vi "Cleanup.vi"(8 "error in (no error)":errorcluster, 11 "PlatformConfigPanel in":refnum<class "PlatformConfigPanel.lvclass">) -> (0 "error out":errorcluster)   [LabVIEW 2020, in "PicoG-App.lvlib" / "PlatformConfigPanel.lvclass"]
uses:
  PlatformConfigPanel.lvclass
  <vilib>/IlluminatedG/IG OOPanel/OOPanel/Panel/Panel.lvclass
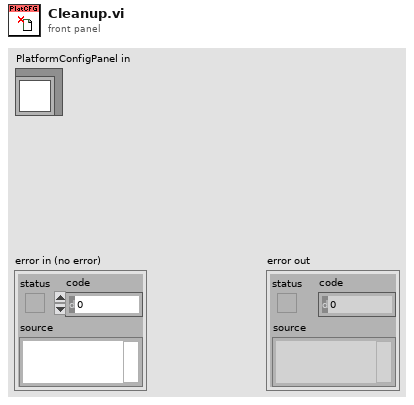
[diagram p1: front panel]
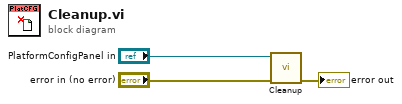
[diagram p0: block diagram]
diagram:
  n1 = call-parent "Cleanup.vi"("error in (no error)"="error in (no error)", "Panel in"="PlatformConfigPanel in") -> ("error out"=→"error out":errorcluster)  [unwired: 9 in]
